vi "LoadProjectList.vi"() -> (0 "Index":i32, 3 "SelectedProject":string)   [LabVIEW 2018]
panel:
  in  "stop":bool
  in  "Cleaned Array":string[](array[string])
  in  "Array":string[](array[string])
  in  "List of project:":string(combo)
  out "ProjectList":string
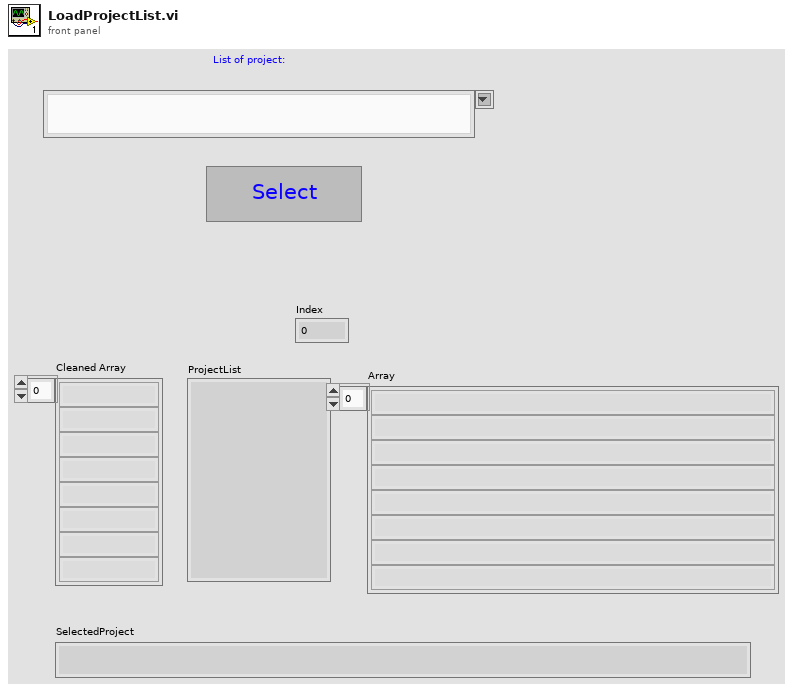
[diagram p1: front panel]
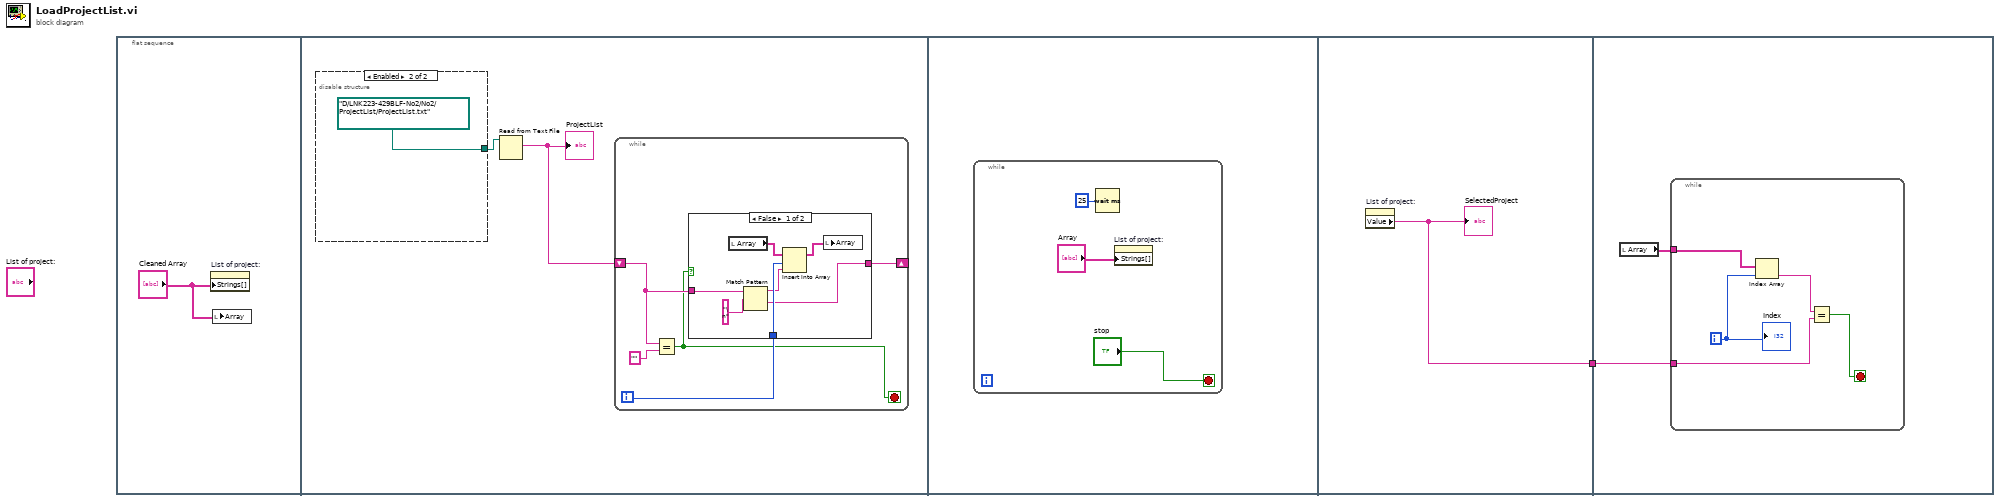
[diagram p0: block diagram]
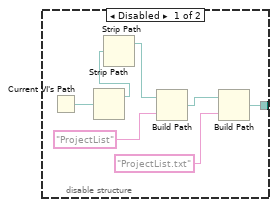
[diagram p2: hidden frame]
diagram:
  n1 = flat-sequence {
    tunnel: [w29] -> w1
    tunnel: w1 -> [w30]
    frame #0 {
      n2 = property on="List of project:" class="CmbBox"("Strings[]"="Cleaned Array") -> ()  [unwired: 2 in, 2 out]
      n3 = local write "Array"("Cleaned Array") -> ()
    }
    frame #1 {
      n4 = disable-structure shown="Enabled" {
        disable-tunnel: [w7 path "D:/LNK223-429BLF-No2/No2/ProjectList/ProjectList.txt" ("appended path")] -> w4
        frame Disabled {
          n5 = Current VI's Path() -> (path=w11:path)
          n6 = Strip Path(path=w11) -> (stripped path=w6:path)  [unwired: 1 out]
          n7 = Strip Path(path=w6) -> (stripped path=w5:path)  [unwired: 1 out]
          n8 = Build Path(base path=w5, name or relative path="ProjectList") -> (appended path=w8:path)
          n9 = Build Path(base path=w8, name or relative path="ProjectList.txt") -> (appended path=w7:path)
        }
        frame Enabled {
        }
      }
      n10 = Read from Text File(file (use dialog)=w4) -> (text=w3:string)  [unwired: 1 in, 5 out]
      "ProjectList" <- w3
      n11 = while {
        shift-right: [w16] -> _
        shift-left: w3 -> [w15]
        i -> [w17]
        stop <- w13 stop-if-true
        n12 = Equal?(x=w15, y="" ("regular expression")) -> (x = y?=w13:bool)
        n13 = case shown="False" w13 {
          tunnel: w17 -> [w22 _]
          tunnel: [w20 w25] -> w16
          tunnel: w15 -> [w19 w25]
          frame False {
            n14 = local read "Array"() -> (w18:string[])
            n15 = Match Pattern(string=w19, regular expression="\n") -> (before substring=w21:string, after substring=w20:string)  [unwired: 3 out]
            n16 = Insert Into Array(array=w18, index=w22, new element=w21) -> (w23:string[])
            n17 = local write "Array"(w23) -> ()
          }
          frame True {
          }
        }
      }
    }
    frame #2 {
      n18 = while {
        stop <- "stop" stop-if-true
        n19 = Wait (ms)(milliseconds to wait=u32 25) -> ()  [unwired: 1 out]
        n20 = property on="List of project:" class="CmbBox"("Strings[]"="Array") -> ()  [unwired: 2 in, 2 out]
      }
    }
    frame #3 {
      n21 = property on="List of project:" class="CmbBox"() -> ("Value"=w29:string)  [unwired: 2 in, 2 out]
      "SelectedProject" <- w29
    }
    frame #4 {
      n22 = local read "Array"() -> (w31:string[])
      n23 = while {
        tunnel: w31 -> [w36]
        tunnel: w30 -> [w33]
        i -> [w35]
        stop <- w32 stop-if-true
        n24 = Index Array(array=w36, index=w35) -> (element=w34:string)
        n25 = Equal?(x=w34, y=w33) -> (x = y?=w32:bool)
        "Index" <- w35
      }
    }
  }
